vi "Append Related Links.vi"(8 "Error In":errorcluster, 10 "Common Related Link(s)":string="learn:libraries:linx:reference:labview:start", 11 "Output Root Directory":path=path "C:/Users/samkristoff/Desktop/Online Help/output/data/pages") -> (0 "Error Out":errorcluster)   [LabVIEW 2014]
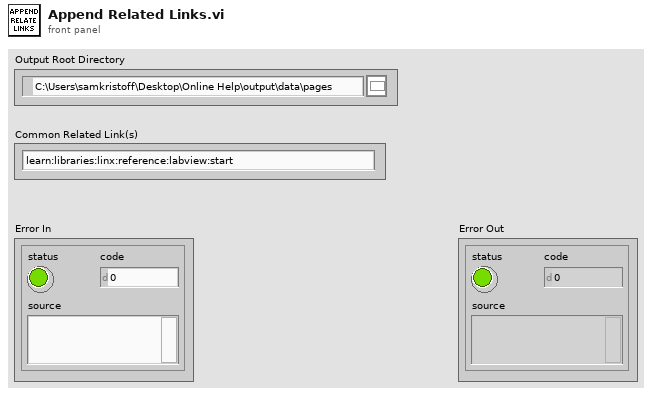
[diagram p1: front panel]
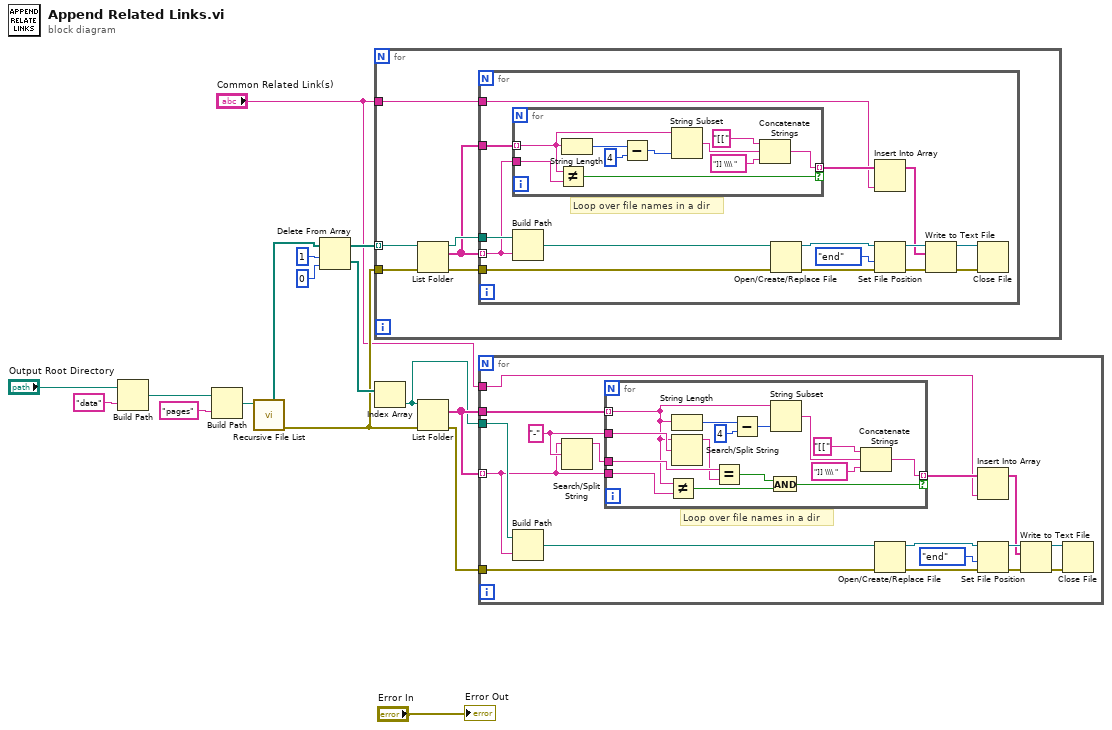
[diagram p0: block diagram]
diagram:
  n1 = Build Path(base path="Output Root Directory", name or relative path="data") -> (appended path=w5:path)
  n2 = Build Path(base path=w5, name or relative path="pages") -> (appended path=w2:path)
  n3 = call <vilib>:"Recursive File List.vi"("Folder Path"=w2) -> ("error out"=w8:errorcluster, "All Folders"=w16:path[])  [unwired: 6 in, 3 out]
  n4 = Delete From Array(array=w16, length=1, index=0) -> (deleted portion=w11:path[], array with subset deleted=w9:path[])
  n5 = for {
    tunnel: w9 -> [w22] mode=indexing
    tunnel: w8 -> [w21]
    tunnel: "Common Related Link(s)" -> [w17]
    n6 = List Folder(path=w22, error in=w21) -> (path out=w20:path, filenames=w18:string[], error out=w19:errorcluster)  [unwired: 2 in, 1 out]
    n7 = for {
      tunnel: w18 -> [w25] mode=indexing
      tunnel: w20 -> [w37]
      tunnel: w19 -> [w28]
      tunnel: w18 -> [w24]
      tunnel: w17 -> [w23]
      # "Loop over file names in a dir"
      n8 = for {
        tunnel: [w41] -> w27 mode=indexing if=w38
        tunnel: w25 -> [w40]
        tunnel: w24 -> [w39] mode=indexing
        n9 = Not Equal?(x=w39, y=w40) -> (x != y?=w38:bool)
        n10 = String Length(string=w39) -> (length=w47:i32)
        n11 = Subtract(x=w47, y=4) -> (x-y=w45:i32)
        n12 = String Subset(string=w39, length (rest)=w45) -> (substring=w44:string)  [unwired: 1 in]
        n13 = Concatenate Strings("[[" ("string"), w44, "]] \\\\ " ("string")) -> (w41:string)
      }
      n14 = Build Path(base path=w37, name or relative path=w25) -> (appended path=w36:path)
      n15 = Open/Create/Replace File(file path (use dialog)=w36, error in=w28) -> (refnum out=w32:refnum<file>, error out=w30:errorcluster)  [unwired: 4 in, 1 out]
      n16 = Insert Into Array(array=w27, new element=w23) -> (w26:string[])  [unwired: 1 in]
      n17 = Set File Position(refnum=w32, from (0:start)=enum16{"start", "end", "current"}."end", error in=w30) -> (refnum out=w33:refnum<file>, error out=w31:errorcluster)  [unwired: 1 in]
      n18 = Write to Text File(file (use dialog)=w33, text=w26, error in=w31) -> (refnum out=w34:refnum<file>, error out=w35:errorcluster)  [unwired: 1 in, 1 out]
      n19 = Close File(refnum=w34, error in=w35) -> ()  [unwired: 2 out]
    }
  }
  n20 = Index Array(array=w11) -> (element=w10:path)  [unwired: 1 in]
  n21 = List Folder(path=w10, error in=w8) -> (filenames=w13:string[], error out=w12:errorcluster)  [unwired: 2 in, 2 out]
  n22 = for {
    tunnel: w13 -> [w49] mode=indexing
    tunnel: w13 -> [w52]
    tunnel: w10 -> [w64]
    tunnel: w12 -> [w55]
    tunnel: "Common Related Link(s)" -> [w48]
    w54 = "-" ("search string/char (-)")
    # "Loop over file names in a dir"
    n23 = Build Path(base path=w64, name or relative path=w49) -> (appended path=w63:path)
    n24 = Search/Split String(string=w49, search string/char (-)=w54) -> (substring before match=w53:string)  [unwired: 1 in, 2 out]
    n25 = for {
      tunnel: w52 -> [w67] mode=indexing
      tunnel: w54 -> [w77]
      tunnel: w53 -> [w79]
      tunnel: [w70] -> w51 mode=indexing if=w65
      tunnel: w49 -> [w68]
      n26 = Not Equal?(x=w67, y=w68) -> (x != y?=w69:bool)
      n27 = String Length(string=w67) -> (length=w76:i32)
      n28 = Search/Split String(string=w67, search string/char (-)=w77) -> (substring before match=w78:string)  [unwired: 1 in, 2 out]
      n29 = Equal?(x=w79, y=w78) -> (x = y?=w66:bool)
      n30 = Subtract(x=w76, y=4) -> (x-y=w74:i32)
      n31 = And(x=w66, y=w69) -> (x .and. y?=w65:bool)
      n32 = String Subset(string=w67, length (rest)=w74) -> (substring=w73:string)  [unwired: 1 in]
      n33 = Concatenate Strings("[[" ("string"), w73, "]] \\\\ " ("string")) -> (w70:string)
    }
    n34 = Open/Create/Replace File(file path (use dialog)=w63, error in=w55) -> (refnum out=w59:refnum<file>, error out=w57:errorcluster)  [unwired: 4 in, 1 out]
    n35 = Insert Into Array(array=w51, new element=w48) -> (w50:string[])  [unwired: 1 in]
    n36 = Set File Position(refnum=w59, from (0:start)=enum16{"start", "end", "current"}."end", error in=w57) -> (refnum out=w60:refnum<file>, error out=w58:errorcluster)  [unwired: 1 in]
    n37 = Write to Text File(file (use dialog)=w60, text=w50, error in=w58) -> (refnum out=w61:refnum<file>, error out=w62:errorcluster)  [unwired: 1 in, 1 out]
    n38 = Close File(refnum=w61, error in=w62) -> ()  [unwired: 2 out]
  }
  "Error Out" <- "Error In"
